vi "cblas dswap.vi"(5 "n":i32=-1, 6 "incy":i32=1, 7 "incx":i32=1, 10 "y":dbl[](array[numeric]), 11 "x":dbl[](array[numeric])) -> (0 "error":i32, 2 "dswap y":dbl[](array[numeric]), 3 "dswap x":dbl[](array[numeric]))   [LabVIEW 2020, in "NI_AALBLAS.lvlib"]
uses:
  <vilib>/Analysis/NI_AALBLAS.lvlib
  <resource>/lvblas.dll
panel:
  # "void cblas_dswap(n, *x, incx, *y, incy)"
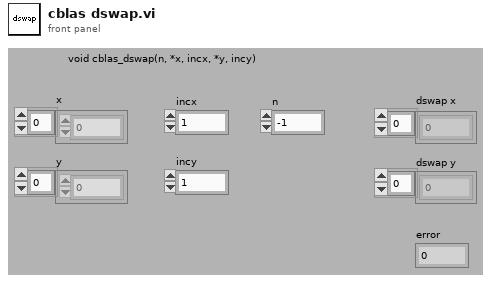
[diagram p1: front panel]
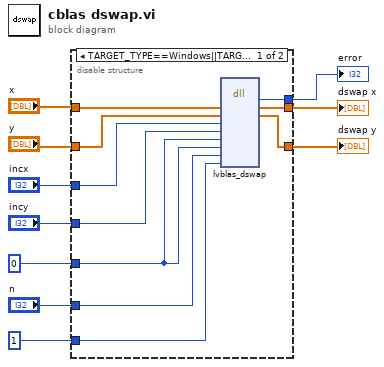
[diagram p0: block diagram]
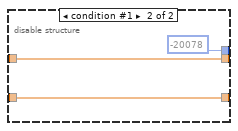
[diagram p2: hidden frame]
diagram:
  n1 = disable-structure shown="TARGET_TYPE==Windows||TARGET_TYPE==Unix||TARGET_TYPE==RT||TARGET_TYPE==Mac" {
    disable-tunnel: "x" -> [w20 w22]
    disable-tunnel: "y" -> [w19 w21]
    disable-tunnel: "n" -> [w18 _]
    disable-tunnel: [w17 -20078] -> w5
    disable-tunnel: [w16 w22] -> w7
    disable-tunnel: [w15 w21] -> w6
    disable-tunnel: 0 -> [w14 _]
    disable-tunnel: "incx" -> [w13 _]
    disable-tunnel: "incy" -> [w12 _]
    disable-tunnel: 1 -> [w11 _]
    frame condition #0 (active) {
      n2 = dll-call lib="e:/builds/penguin/labview/branches/2020/dev/dist/resource/lvblas.*" fn="lvblas_dswap" ("CBLAS.dll:DotProdH")("X"=w20, "Y"=w19, "IncX"=w13, "IncY"=w12, "startX"=w14, "startY"=w14, "N"=w18, "check"=w11) -> ("error"=w17:i32, "X"=w16:dbl[], "Y"=w15:dbl[])  [unwired: 9 in, 2 out]
    }
    frame condition #1 {
    }
  }
  "error" <- w5
  "dswap x" <- w7
  "dswap y" <- w6
